vi "Evaluate Status.vi"(11 "Statuses":T1[](array[typedef])) -> (3 "Status":T1=enum."Passed")   [LabVIEW 2020, in "Result Model.lvclass"]
uses:
  Result Model.lvclass
  Core/Result/Status.ctl
  Core/Result/Result.lvlib
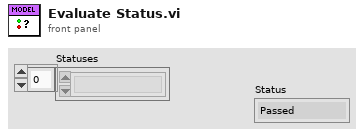
[diagram p1: front panel]
types:
  T1 = typedef "Result.lvlib/Status.ctl" = enum16{"", "Passed", "Failed", "Error", "Skipped", "Setup Error", "Broken", "Teardown Error"}
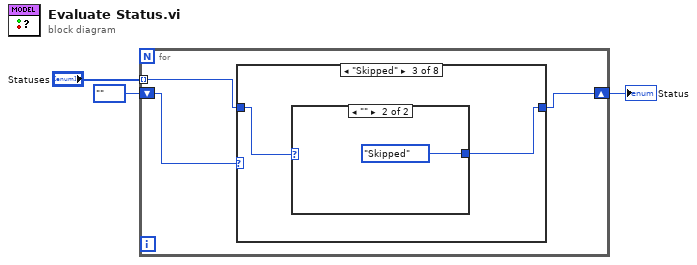
[diagram p0: block diagram]
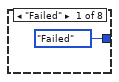
[diagram p3: hidden frame]
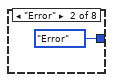
[diagram p4: hidden frame]
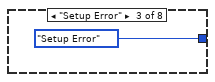
[diagram p5: hidden frame]
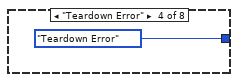
[diagram p6: hidden frame]
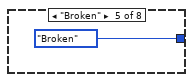
[diagram p7: hidden frame]
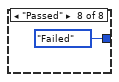
[diagram p9: hidden frame]
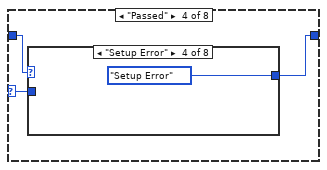
[diagram p12: hidden frame]
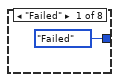
[diagram p13: hidden frame]
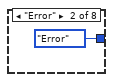
[diagram p14: hidden frame]
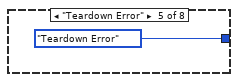
[diagram p16: hidden frame]
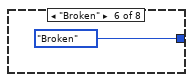
[diagram p17: hidden frame]
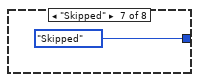
[diagram p18: hidden frame]
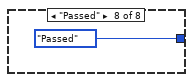
[diagram p19: hidden frame]
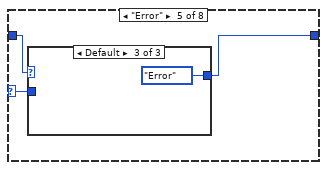
[diagram p20: hidden frame]
diagram:
  n1 = for {
    tunnel: "Statuses" -> [w4] mode=indexing
    shift-right: [w5] -> w2
    shift-left: Status."" ("Current") -> [w6]
    n2 = case shown="\"Skipped\"" w6 {
      selector: w6 -> [w7 _ _ w23 w34 _ _ _]
      tunnel: w4 -> [w9 w18 w19 w25 w35 w40 w44 w48]
      tunnel: [w8 w18 w20 w24 w36 w41 w45 w49] -> w5
      frame "Failed" {
        n3 = case shown="\"\"" w9 {
          tunnel: [Status."Failed" ("Merged Status") Status."Error" ("Merged Status") Status."Setup Error" ("Merged Status") Status."Teardown Error" ("Merged Status") Status."Broken" ("Merged Status") w15 w16 Status."Failed" ("Merged Status")] -> w8
          tunnel: w7 -> [_ _ _ _ _ w15 w16 _]
          frame "Failed" {
          }
          frame "Error" {
          }
          frame "Setup Error" {
          }
          frame "Teardown Error" {
          }
          frame "Broken" {
          }
          frame "" {
          }
          frame "Skipped" {
          }
          frame "Passed" {
          }
        }
      }
      frame "" {
      }
      frame "Skipped" {
        n4 = case shown="\"\"" w19 {
          selector: w19 -> [w21 _]
          tunnel: [w21 Status."Skipped" ("Merged Status")] -> w20
          frame Default {
          }
          frame "" {
          }
        }
      }
      frame "Passed" {
        n5 = case shown="\"Setup Error\"" w25 {
          tunnel: [Status."Failed" ("Merged Status") Status."Error" ("Merged Status") w28 Status."Setup Error" ("Merged Status") Status."Teardown Error" ("Merged Status") Status."Broken" ("Merged Status") Status."Skipped" ("Merged Status") Status."Passed" ("Merged Status")] -> w24
          tunnel: w23 -> [_ _ w28 _ _ _ _ _]
          frame "Failed" {
          }
          frame "Error" {
          }
          frame "" {
          }
          frame "Setup Error" {
          }
          frame "Teardown Error" {
          }
          frame "Broken" {
          }
          frame "Skipped" {
          }
          frame "Passed" {
          }
        }
      }
      frame "Error" {
        n6 = case shown="Default" w35 {
          tunnel: [Status."Skipped" ("Merged Status") w38 Status."Error" ("Merged Status")] -> w36
          tunnel: w34 -> [_ w38 _]
          frame "Skipped" {
          }
          frame "" {
          }
          frame Default {
          }
        }
      }
      frame "Setup Error" {
        n7 = case shown="Default" w40 {
          tunnel: [Status."Skipped" ("Merged Status") Status."Setup Error" ("Merged Status")] -> w41
          frame "Skipped" {
          }
          frame Default {
          }
        }
      }
      frame "Broken" {
        n8 = case shown="Default" w44 {
          tunnel: [Status."Broken" ("Merged Status") Status."Setup Error" ("Merged Status")] -> w45
          frame Default {
          }
          frame "Setup Error" {
          }
        }
      }
      frame "Teardown Error" {
        n9 = case shown="Default" w48 {
          tunnel: [Status."Skipped" ("Merged Status") Status."Teardown Error" ("Merged Status")] -> w49
          frame "Skipped" {
          }
          frame Default {
          }
        }
      }
    }
  }
  "Status" <- w2
